vi "Read_Net_Var.vi"(11 "Array 2":refnum<k21>[](array[refnum])=["ni.var.psp://iv/Impedance Bridge/Temperature B", "ni.var.psp://iv/Impedance Bridge/Temperature C", "ni.var.psp://iv/Impedance Bridge/Temperature D", "ni.var.psp://iv/Impedance Bridge/Temperature E"]) -> (3 "Array":dbl[](array[numeric]))   [LabVIEW 2013]
panel:
  in  "stop":bool
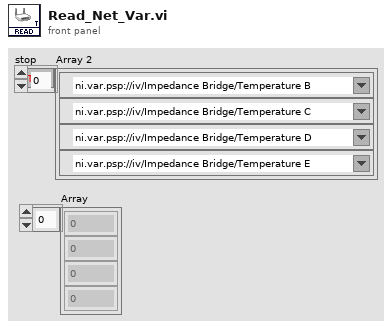
[diagram p1: front panel]
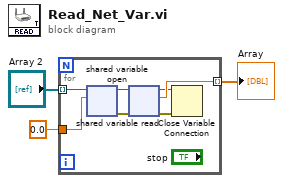
[diagram p0: block diagram]
diagram:
  n1 = for {
    tunnel: 0.0 -> [w8]
    tunnel: [w7] -> w2 mode=indexing
    tunnel: "Array 2" -> [w6] mode=indexing
    n2 = shared-variable-open(w6, w8) -> (w10:refnum<k21>, w9:errorcluster)  [unwired: 2 in]
    n3 = shared-variable-read(w10, w9) -> (w5:refnum<k21>, w4:errorcluster, w7:dbl)  [unwired: 1 out]
    n4 = Close Variable Connection(8:w4, 11:w5) -> ()  [unwired: 1 out]
  }
  "Array" <- w2
